vi "CANOpen RPDO Channel.vi"(8 "error in (no error)":errorcluster, 11 "Node Ptr":T3 format="%.0x") -> (0 "error out":errorcluster)   [LabVIEW 2013, in "CANOpen Addon Custom Device.lvlib"]
uses:
  CANOpen Addon Custom Device.lvlib
  <vilib>/NI Veristand/Custom Device API/Custom Device Item Ref.ctl
  Shared Code/CANOpen_PDO Data Type.ctl
  SubVIs/CANopen Byte Order.ctl
  Shared Code/CANOpen Addon GUID Lookup Global.vi
  <vilib>/NI Veristand/Custom Device API/Get Item Property (Variant).vi
  <vilib>/NI Veristand/Custom Device API/Set Item Property (Variant).vi
  <vilib>/NI Veristand/Custom Device API/Custom Device API.lvlib
panel:
  in  "Default Value":dbl
  in  "*Byte Order":T1=enum."little-endian" caption="Byte Order"
  in  "*Bit Offset":u8 caption="Bit Offset" max=8 step=1
  in  "SHDocVw.IWebBrowser2":refnum<k7>(container)
  in  "*Data Type":T2 caption="Data Type"
  in  "*Byte Offset":u8 caption="Byte Offset" max=8 step=1
  in  "*Scale Offset":dbl caption="Scale Offset"
  in  "*Scale Factor":dbl caption="Scale Factor"
  in  "Header":cluster{"Section Name":string}={"Section Name"="RPDO"}
  in  "Description":string
  in  "Parameter Name":string
  # "CANopen send value = (NI VeriStand channel value - Scale Offset) / Scale Factor"
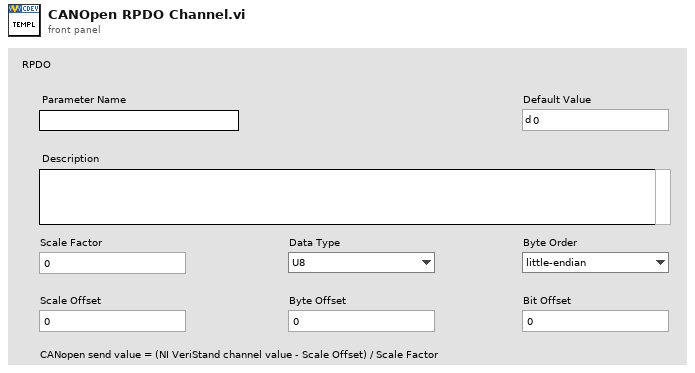
[diagram p1: front panel]
types:
  T1 = typedef "CANOpen Addon Custom Device.lvlib/CANopen Byte Order.ctl" = enum16{"big-endian network order", "little-endian"}
  T2 = typedef "CANOpen Addon Custom Device.lvlib/CANOpen_PDO Data Type.ctl" = enum16{"U8", "U16", "U32", "I8", "I16", "I32", "Single", "Double", "Boolean"}
  T3 = typedef "Custom Device API.lvlib/Custom Device Item Ref.ctl" = u64
  T4 = typedef "Custom Device API.lvlib/Custom Device Channel.ctl" = cluster{"Type":T5, "Units":string, "Default Value":dbl, "Faultable":bool, "Scalable":bool}
  T5 = typedef "Custom Device API.lvlib/Custom Device Channel Type.ctl" = enum16{"Input", "Output"}
  T6 = typedef "Custom Device API.lvlib/Custom Device Item Info.ctl" = cluster{"Name":string, "Is Channel":bool, "GUID":string, "Is Waveform":bool}
  T7 = typedef "Custom Device API.lvlib/Custom Device Commands.ctl" = enum16{"Default", "Item renamed", "Shutdown", "Dynamic button pressed"}
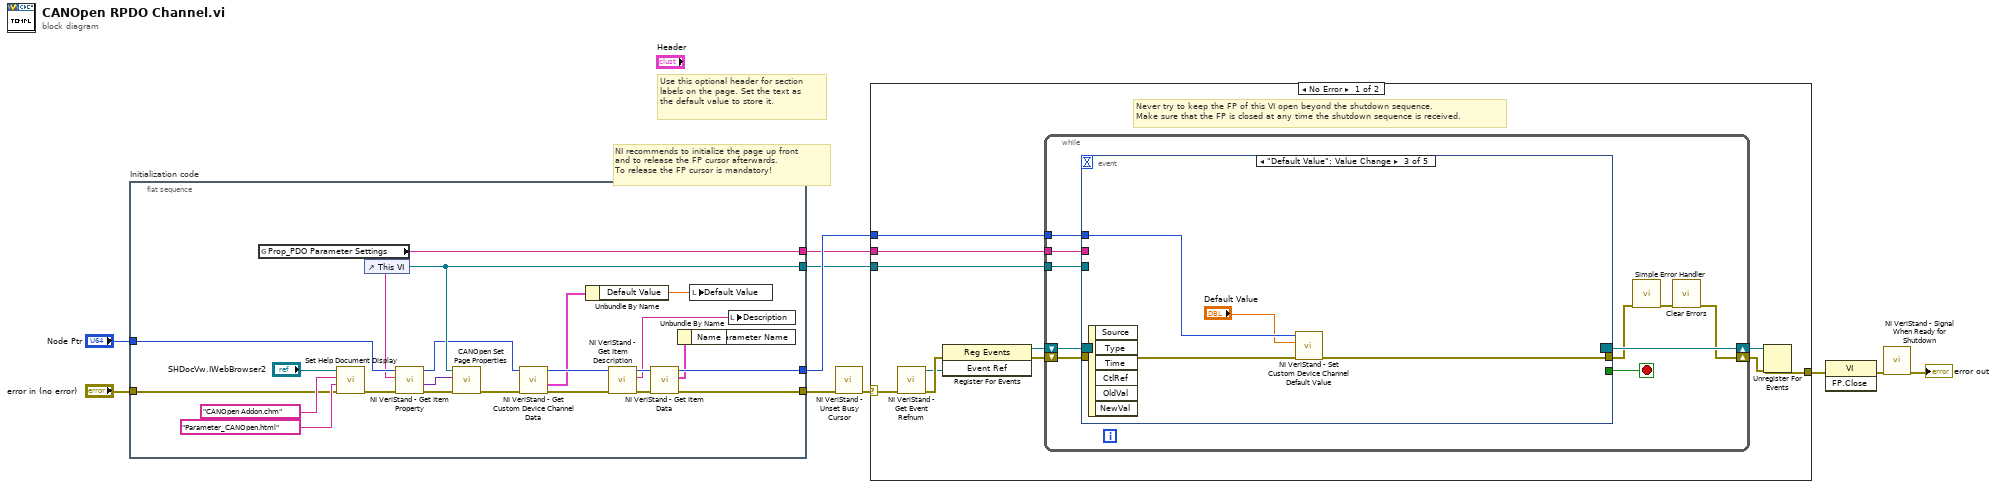
[diagram p0: block diagram]
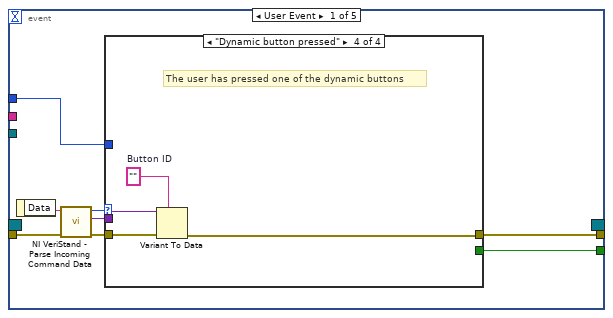
[diagram p2: hidden frame]
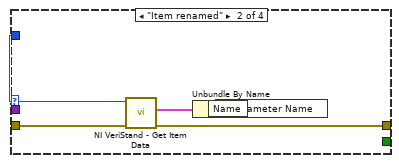
[diagram p4: hidden frame]
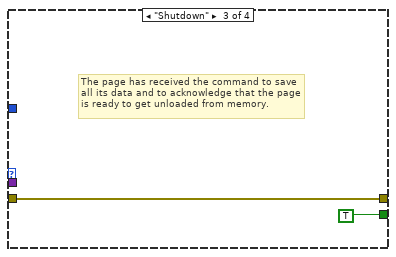
[diagram p5: hidden frame]
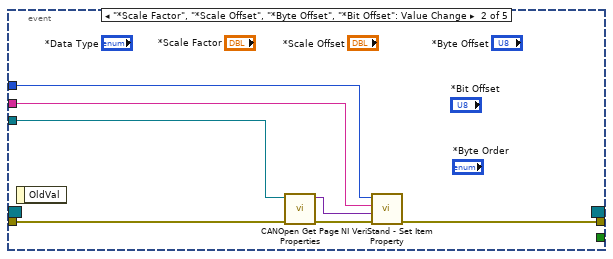
[diagram p6: hidden frame]
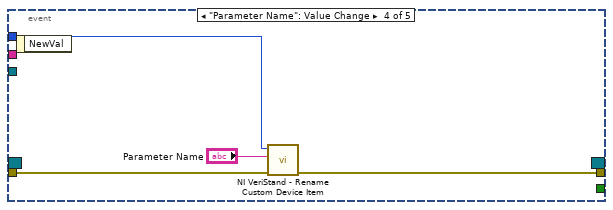
[diagram p7: hidden frame]
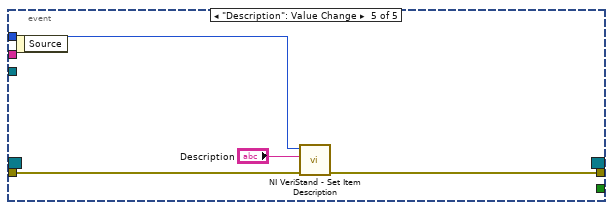
[diagram p8: hidden frame]
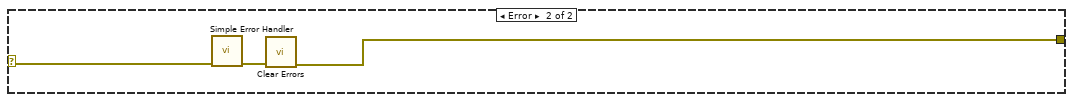
[diagram p9: hidden frame]
diagram:
  # "Use this optional header for section labels on the page. Set the text as the default value to store it."
  # "NI recommends to initialize the page up front\nand to release the FP cursor afterwards.\nTo release the FP cursor is mandatory!"
  n1 = flat-sequence "Initialization code" {
    tunnel: "error in (no error)" -> [w21]
    tunnel: "Node Ptr" -> [w19]
    tunnel: [w27] -> w6
    tunnel: [w33] -> w3
    tunnel: [w18] -> w2
    tunnel: [w17] -> w1
    frame #0 {
      n2 = global read "CANOpen Addon GUID Lookup Global.vi" "Prop_PDO Parameter Settings"() -> (w17:string)
      n3 = call "Set Help Document Display.vi"("error in (no error)"=w21, "HTML File"="Parameter_CANOpen.html", "Main CHM File"="CANOpen Addon.chm", "SHDocVw.IWebBrowser2"="SHDocVw.IWebBrowser2") -> ("error out"=w23:errorcluster)  [unwired: 7 in]
      n4 = control-ref of="This VI"() -> (w18:refnum<vi>)
      n5 = call-poly <vilib>:"NI VeriStand - Get Item Property.vi"("error in (no error)"=w23, "Property Name"=w17, "Item Ref in"=w19) -> ("error out"=w20:errorcluster, "Value"=w22:variant, "Item Ref out"=w14:T3)  [unwired: 5 in, 1 out]
      n6 = call "CANOpen Set Page Properties.vi"("error in"=w20, "variant"=w22, "This VI"=w18) -> ("error out"=w16:errorcluster)  [unwired: 8 in]
      n7 = call <vilib>:"NI VeriStand - Get Custom Device Channel Data.vi"("error in (no error)"=w16, "Channel Ref in"=w14) -> ("error out"=w15:errorcluster, "Channel"=w12:T4, "Channel Ref out"=w13:T3)  [unwired: 7 out]
      n8 = Unbundle By Name(w12) -> ("Default Value"=w11:dbl)
      n9 = call <vilib>:"NI VeriStand - Get Item Description.vi"("error in (no error)"=w15, "Item Ref in"=w13) -> ("error out"=w30:errorcluster, "Description"=w31:string, "Item Ref out"=w32:T3)  [unwired: 7 out]
      n10 = call <vilib>:"NI VeriStand - Get Item Data.vi"("error in (no error)"=w30, "Item Ref in"=w32) -> ("error out"=w27:errorcluster, "Item Info"=w29:T6, "Item Ref out"=w33:T3)  [unwired: 7 out]
      n11 = Unbundle By Name(w29) -> ("Name"=w28:string)
      n12 = local write "Default Value"(w11) -> ()
      n13 = local write "Parameter Name"(w28) -> ()
      n14 = local write "Description"(w31) -> ()
    }
  }
  n15 = call <vilib>:"NI VeriStand - Unset Busy Cursor.vi"("error in (no error)"=w6) -> ("error out"=w5:errorcluster)  [unwired: 10 out]
  n16 = case shown="No Error" w5 {
    selector: w5 -> [w36 w96]
    tunnel: [w41 w94] -> w10
    tunnel: w3 -> [w37 _]
    tunnel: w2 -> [w35 _]
    tunnel: w1 -> [w34 _]
    frame No Error {
      # "Never try to keep the FP of this VI open beyond the shutdown sequence.\nMake sure that the FP is closed at any time the shutdown sequence is received."
      n17 = call <vilib>:"NI VeriStand - Get Event Refnum.vi"("error in (no error)"=w36) -> ("error out"=w44:errorcluster, "Event Ref"=w40:refnum<user-event>)  [unwired: 9 out]
      n18 = register-events(error in=w44, w40) -> (reference out=w38:refnum<event-registration>, error out=w39:errorcluster)  [unwired: 1 in]
      n19 = while {
        tunnel: w37 -> [w50]
        shift-right: [w47] -> w42
        shift-left: w39 -> [w53]
        shift-right: [w54] -> w43
        shift-left: w38 -> [w52]
        tunnel: w35 -> [w46]
        tunnel: w34 -> [w45]
        stop <- w51 stop-if-true
        n20 = event shown="[2] \"Default Value\": Value Change" {
          selector: w52 -> [_ _ _ _ _]
          dyn-events: [_ _ _ _ _] -> w54
          timeout: _ -> [_ _ _ _ _]
          tunnel: w53 -> [w62 w81 w85 w89 w92]
          tunnel: [w58 _ _ _ _] -> w51
          tunnel: [w57 w78 w82 w88 w91] -> w49
          tunnel: w50 -> [w56 w76 w84 w87 w93]
          tunnel: w46 -> [_ w80 _ _ _]
          tunnel: w45 -> [_ w75 _ _ _]
          event User Event {
            n21 = event-data() -> ("Data"=w61:string)  [unwired: 1 out]
            n22 = call <vilib>:"NI VeriStand - Parse Incoming Command Data.vi"("error in (no error)"=w62, "Incoming data"=w61) -> ("error out"=w60:errorcluster, "Outgoing data"=w55:variant, "Action"=w59:T7)  [unwired: 7 out]
            n23 = case shown="\"Dynamic button pressed\"" w59 {
              tunnel: w60 -> [w63 w68 w69 w74]
              tunnel: [_ _ TRUE _] -> w58
              tunnel: [w63 w65 w69 w71] -> w57
              tunnel: w56 -> [_ w67 _ _]
              tunnel: w55 -> [_ _ _ w73]
              frame "Default", Default {
              }
              frame "Item renamed" {
                n24 = call <vilib>:"NI VeriStand - Get Item Data.vi"("error in (no error)"=w68, "Item Ref in"=w67) -> ("error out"=w65:errorcluster, "Item Info"=w66:T6)  [unwired: 8 out]
                n25 = Unbundle By Name(w66) -> ("Name"=w64:string)
                n26 = local write "Parameter Name"(w64) -> ()
              }
              frame "Shutdown" {
                # "The page has received the command to save all its data and to acknowledge that the page is ready to get unloaded from memory."
              }
              frame "Dynamic button pressed" {
                w72 = ""  # Button ID
                # "The user has pressed one of the dynamic buttons"
                n27 = Variant To Data(error in=w74, type=w72, Variant=w73) -> (error out=w71:errorcluster)  [unwired: 1 out]
              }
            }
          }
          event "*Scale Factor", "*Scale Offset", "*Byte Offset", "*Bit Offset": Value Change {
            n28 = event-data() -> ()  [unwired: 2 out]
            n29 = call "CANOpen Get Page Properties.vi"("error in (no error)"=w81, "This VI"=w80) -> ("error out"=w79:errorcluster, "Settings"=w77:variant)  [unwired: 8 in]
            n30 = call-poly <vilib>:"NI VeriStand - Set Item Property.vi"("error in (no error)"=w79, "Value"=w77, "Property Name"=w75, "Item Ref in"=w76) -> ("error out"=w78:errorcluster)  [unwired: 5 in, 2 out]
          }
          event "Default Value": Value Change {
            n31 = event-data() -> ()  [unwired: 7 out]
            n32 = call <vilib>:"NI VeriStand - Set Custom Device Channel Default Value.vi"("error in (no error)"=w85, "Default Value"="Default Value", "Channel Ref in"=w84) -> ("error out"=w82:errorcluster)  [unwired: 7 in, 1 out]
          }
          event "Parameter Name": Value Change {
            n33 = event-data() -> ()  [unwired: 2 out]
            n34 = call <vilib>:"NI VeriStand - Rename Custom Device Item.vi"("error in (no error)"=w89, "New Name"="Parameter Name", "Item Ref in"=w87) -> ("error out"=w88:errorcluster)  [unwired: 1 in, 7 out]
          }
          event "Description": Value Change {
            n35 = event-data() -> ()  [unwired: 2 out]
            n36 = call <vilib>:"NI VeriStand - Set Item Description.vi"("error in (no error)"=w92, "Description"="Description", "Item Ref in"=w93) -> ("error out"=w91:errorcluster)  [unwired: 8 out]
          }
        }
        n37 = call <vilib>:"Simple Error Handler.vi"("error in (no error)"=w49) -> ("error out"=w48:errorcluster)  [unwired: 1 in, 7 out]
        n38 = call <vilib>:"Clear Errors.vi"("error in (no error)"=w48) -> ("error out"=w47:errorcluster)  [unwired: 6 out]
      }
      n39 = Unregister For Events(event registration refnum=w43, error in=w42) -> (error out=w41:errorcluster)
    }
    frame Error {
      n40 = call <vilib>:"Simple Error Handler.vi"("error in (no error)"=w96) -> ("error out"=w95:errorcluster)  [unwired: 1 in, 7 out]
      n41 = call <vilib>:"Clear Errors.vi"("error in (no error)"=w95) -> ("error out"=w94:errorcluster)  [unwired: 6 out]
    }
  }
  n42 = invoke class="VI" method="FP.Close"(error in=w10) -> (error out=w9:errorcluster)  [unwired: 2 in, 2 out]
  n43 = call <vilib>:"NI VeriStand - Signal When Ready for Shutdown.vi"("error in (no error)"=w9) -> ("error out"=→"error out":errorcluster)  [unwired: 10 out]
